vi "ProcessRequest.vi"(6 "CustomMessage":string, 8 "ErrorIn":errorcluster, 9 "RequestType":T2, 11 "DeviceResourceName":refnum<visa-resource-name>) -> (0 "ErrorOut":errorcluster, 2 "BytesReadNr":u32, 3 "Response":string, 5 "Request":T1={"Type"=enum."Reset", "Command"="", "Mode"={"Direction"=enum."TransmitOnly", "BytesToRead"=0}} {"Mode"."BytesToRead" min=1 max=4000000000 step=1})   [LabVIEW 2016]
doc: "Communicate with Fall Sensor. All available requests are defined by FindRequestByType SubVI. Warning: this VI requires established connection via Serial COM port before execution. Basic master-slave functionality: send request to device, get response."
uses:
  Requests/RequestType.ctl
  Requests/Request.ctl
  FTDI/COMMode.ctl
  FTDI/COMDirection.ctl
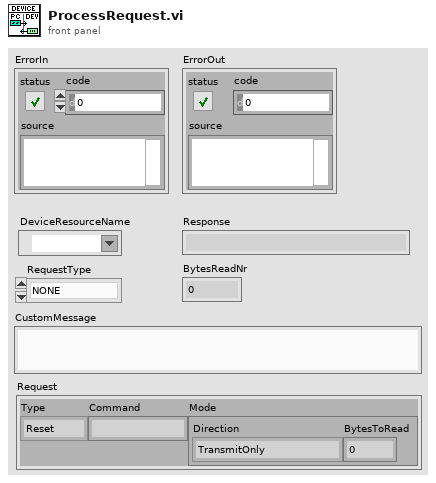
[diagram p1: front panel]
types:
  T1 = typedef "Request.ctl" = cluster{"Type":T2, "Command":string, "Mode":T3}
  T2 = typedef "RequestType.ctl" = enum16{"NONE", "Reset", "Hello", "GetPacketsNr", "GetPacket", "GetConfig", "SetConfig", "SendConfig", "Goodbye"}
  T3 = typedef "COMMode.ctl" = cluster{"Direction":T4, "BytesToRead":u32}
  T4 = typedef "COMDirection.ctl" = enum16{"CommandAndResponse", "ReceiveOnly", "TransmitOnly", "CustomMessageAndResponse"}
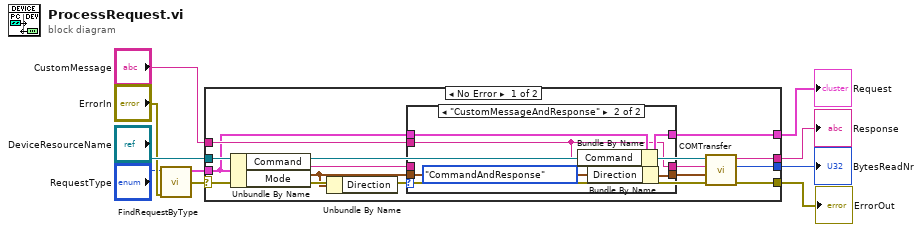
[diagram p0: block diagram]
diagram:
  n1 = call "FindRequestByType.vi"("ErrorIn"="ErrorIn", "RequestType"="RequestType") -> ("ErrorOut"=w10:errorcluster, "Request"=w9:T1)  [unwired: 8 in]
  n2 = case shown="No Error" w10 {
    selector: w10 -> [w22 w34]
    tunnel: w9 -> [w16 w33]
    tunnel: "DeviceResourceName" -> [w23 _]
    tunnel: [w21 _] -> w7
    tunnel: [w20 _] -> w6
    tunnel: [w19 w34] -> w5
    tunnel: [w11 w33] -> w4
    tunnel: "CustomMessage" -> [w17 _]
    frame No Error {
      n3 = Unbundle By Name(w16) -> ("Command"=w15:string, "Mode"=w12:T3)
      n4 = Unbundle By Name(w12) -> ("Direction"=w18:T4)
      n5 = case shown="\"CustomMessageAndResponse\"" w18 {
        tunnel: w17 -> [_ w27]
        tunnel: w16 -> [w24 w29]
        tunnel: w15 -> [w26 _]
        tunnel: [w26 w27] -> w14
        tunnel: [w25 w31] -> w13
        tunnel: w12 -> [w25 w32]
        tunnel: [w24 w28] -> w11
        frame Default {
        }
        frame "CustomMessageAndResponse" {
          n6 = Bundle By Name(cluster=w29, "Command"=w27) -> (w28:T1)
          n7 = Bundle By Name(cluster=w32, "Direction"=COMDirection."CommandAndResponse") -> (w31:T3)
        }
      }
      n8 = call "COMTransfer.vi"("ErrorIn"=w22, "Mode"=w13, "Command"=w14, "Refnum"=w23) -> ("ErrorOut"=w19:errorcluster, "BytesReadNr"=w20:u32, "Response"=w21:string)  [unwired: 5 in]
    }
    frame Error {
    }
  }
  "Response" <- w7
  "BytesReadNr" <- w6
  "ErrorOut" <- w5
  "Request" <- w4
